vi "Close All Bus Monitors.vi"(11 "MonitoredMediator in":refnum<class "MonitoredMediator.lvclass">) -> (3 "MonitoredMediator out":refnum<class "MonitoredMediator.lvclass">)   [LabVIEW 2018, in "MVA Framework.lvlib" / "MonitoredMediator.lvlib" / "MonitoredMediator.lvclass"]
uses:
  MonitoredMediator.lvclass
  IBusMonitor/IBusMonitor.lvclass
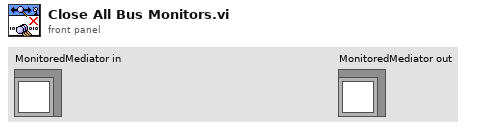
[diagram p1: front panel]
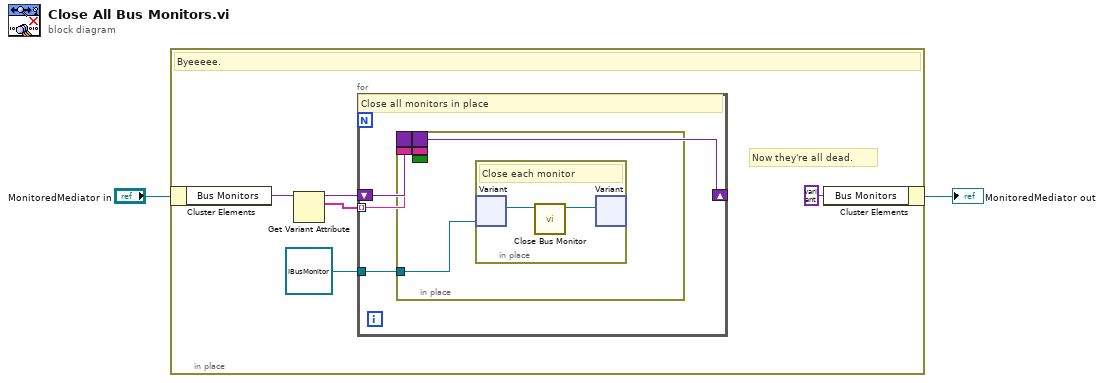
[diagram p0: block diagram]
diagram:
  n1 = in-place {
    # "Now they're all dead."
    # "Byeeeee."
    n2 = in-place-cluster #1("MonitoredMediator in") -> ("Bus Monitors"=w7:variant)
    n3 = Get Variant Attribute(Variant=w7) -> (duplicate Variant=w6:variant, names=w5:string[])  [unwired: 3 in, 2 out]
    n4 = for {
      shift-right: [w8] -> _
      shift-left: w6 -> [w11]
      tunnel: w5 -> [w10] mode=indexing
      tunnel: refnum<class "IBusMonitor.lvclass"> refnum ("MonitoredMediator.lvlib:IBusMonitor.lvclass") -> [w9]
      # "Close all monitors in place"
      n5 = in-place {
        border: w11 -> [_]
        border: w10 -> [_]
        border: [_] -> w8
        border: _ -> [_]
        border: _ -> [_]
        in-place-border: w9 -> [w13]
        n6 = in-place {
          # "Close each monitor"
          n7 = in-place-variant #2(w14, w13) -> (w16:refnum<class "IBusMonitor.lvclass">)  [unwired: 1 out]
          n8 = call-dynamic "Close Bus Monitor.vi"("IBusMonitor In"=w16) -> ("IBusMonitor Out"=w15:refnum<class "IBusMonitor.lvclass">)  [unwired: 10 in]
          n9 = in-place-variant #2(w15) -> (w12:variant)  [unwired: 1 out]
        }
      }
    }
    n10 = in-place-cluster #1("Bus Monitors"=variant ("Active Bus Monitors")) -> (→"MonitoredMediator out":refnum<class "MonitoredMediator.lvclass">)
  }
